vi "Test_Draw_ARGB_With_Mask.vi"(8 "error in (no error)":errorcluster, 11 "Test Case In":refnum<class "Image.lvclass">) -> (0 "error out":errorcluster, 3 "Test Case Out":refnum<class "Image.lvclass">)   [LabVIEW 2020, in "g_ar_toolkit.test.lvlib" / "Image.lvclass"]
uses:
  Image.lvclass
  C:/Program Files (x86)/National Instruments/LabVIEW 2020/vi.lib/Astemes/LUnit/Test Case.lvclass
  g_ar_toolkit.image/Image Size (Fixed).ctl
  <vilib>/Astemes/LUnit/Test Case.lvclass/Test Case.ctl
  g_ar_toolkit.image/CreateEmptyImageGreyscale.vi
  g_ar_toolkit.image/CreateEmptyImageARGB.vi
  g_ar_toolkit.image/CopyPixmapToImageOuptutMaskARGB.vi
  g_ar_toolkit.image/DrawImageWithMaskToPictureARGB.vi
  4993e8ee-a06a-463a-9684-69129f64d5ce.vi
  g_ar_toolkit.image/CreateEmptyImageGreyscale.vi/6598b9e0-8a08-46f5-91fd-ca1b87217137.vi
  g_ar_toolkit.image/CreateEmptyImageARGB.vi/3321fa97-f432-4e1e-8db9-a0df79aed21b.vi
  g_ar_toolkit.image/CopyPixmapToImageOuptutMaskARGB.vi/80b1166a-8c06-443b-b271-eb6a715622f7.vi
  g_ar_toolkit.image/DrawImageWithMaskToPictureARGB.vi/8cd07b1b-062e-4fe4-9e87-2eb3dc89fe0e.vi
  <vilib>/Astemes/LUnit/Append Pass Result.vi
  <vilib>/Astemes/LUnit/Append Fail Result.vi
  <vilib>/Astemes/LUnit/Describe Comparison.vi
  <vilib>/Astemes/LUnit/Compare Variants.vi
  g_ar_toolkit.image/FixPixmapColourArraySize.vi
  <vilib>/Astemes/LUnit/Variant to string.vi
  g_ar_toolkit.image/Default8bitColourMap.vi
  g_ar_toolkit.image/ARGBColourToU32.vi
  <vilib>/Utility/error.llb/Error Cluster From Error Code.vi
  <vilib>/picture/picture.llb/Draw Rectangle.vi
  <vilib>/picture/pictutil.llb/Picture to Pixmap.vi
  <vilib>/Utility/Data Type/Get Type Information.vi
  <vilib>/Utility/LVClass/Get LV Class Name.vi
  Image.lvclass/Image.ctl
  g_ar_toolkit.image/g_ar_toolkit.image.lvlib
panel:
  out "Actual":picture
  out "Expected":picture
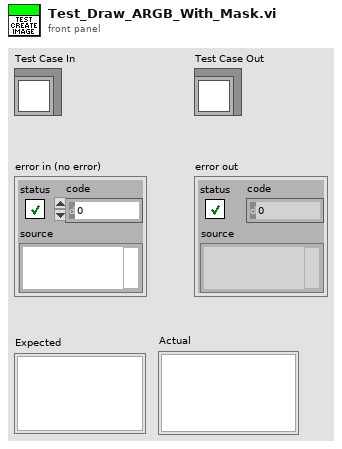
[diagram p1: front panel]
types:
  T1 = typedef "g_ar_toolkit.image.lvlib/Image Size (Fixed).ctl" = cluster{"Width":u16, "Height":u16}
  T2 = typedef "imagedata.ctl" = cluster{"image type":i32, "image depth":i32, "image":u8[], "mask":u8[], "colors":u32[], "Rectangle":cluster{"left":i16, "top":i16, "right":i16, "bottom":i16}}
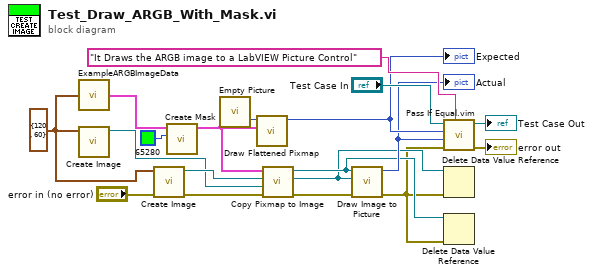
[diagram p0: block diagram]
diagram:
  w4 = T1 {"Width"=120, "Height"=60} ("Preallocated Image Size (Default - 0,0)")
  n1 = call "ExampleARGBImageData.vi"("Image Size"=w4) -> ("RGB Image Data"=w11:T2)
  n2 = call-poly "Create Image.vi"("Preallocated Image Size (Default 0,0)"=w4) -> ("New Greyscale Image"=w7:refnum<data-value>)  [unwired: 9 in, 1 out]
  n3 = call-poly "Create Image.vi"("error in (no error)"="error in (no error)", "Preallocated Image Size (Default: 0,0)"=w4) -> ("error out"=w9:errorcluster, "New ARGB Image"=w8:refnum<data-value>)  [unwired: 8 in]
  n4 = call <vilib>:"Create Mask.vi"("Mask Color (Black)"=u32 65280, "image data"=w11) -> ("image data"=w5:T2)  [unwired: 9 in]
  n5 = call "Empty Picture"() -> ("empty picture"=w14:picture)
  n6 = call <vilib>:"Draw Flattened Pixmap.vi"("image data"=w5, "picture"=w14) -> ("new picture"=w13:picture)  [unwired: 7 in]
  "Expected" <- w13
  n7 = call-poly "Copy Pixmap to Image.vi"("error in (no error)"=w9, "Greyscale Image Mask"=w7, "ARGB Image Destination"=w8, "Pixmap Image Data"=w5) -> ("error out"=w6:errorcluster, "Greyscale Image Mask (duplicate)"=w2:refnum<data-value>, "ARGB Image Destination (duplicate)"=w3:refnum<data-value>)  [unwired: 5 in]
  n8 = call-poly "Draw Image to Picture.vi"("error in (no error)"=w6, "Greyscale Mask"=w2, "ARGB Image Source"=w3) -> ("error out"=w1:errorcluster, "Picture"=w12:picture)  [unwired: 7 in]
  "Actual" <- w12
  n9 = call "Pass If Equal.vim"("Description"="It Draws the ARGB image to a LabVIEW Picture Control", "error in (no error)"=w1, "Actual"=w12, "Expected"=w13, "LUnit Test Case In"="Test Case In") -> ("error out"=→"error out":errorcluster, "LUnit Test Case Out"=→"Test Case Out":refnum<class "Image.lvclass">)  [unwired: 5 in]
  n10 = Delete Data Value Reference(data value reference=w2, error in=w1) -> ()  [unwired: 2 out]
  n11 = Delete Data Value Reference(data value reference=w3, error in=w1) -> ()  [unwired: 2 out]
